vi "check unsalvageable connection.vi"(8 "error in (no error)":errorcluster, 11 "connection reference":refnum<data-value>) -> (0 "error out":errorcluster)   [LabVIEW 2015, in "SubVIs.lvlib" / "TCP Slave.lvclass"]
uses:
  <vilib>/Modbus/subvis/Protocol/TCP/TCP Slave/TCP Slave.lvclass
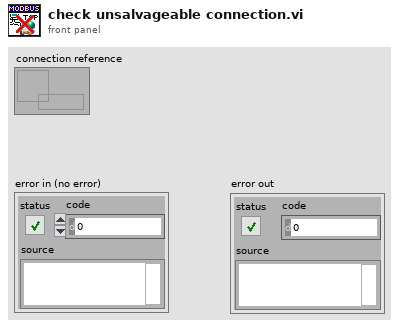
[diagram p1: front panel]
types:
  T1 = cluster{"Connected?":bool, "IP address":string, "connection error":errorcluster}
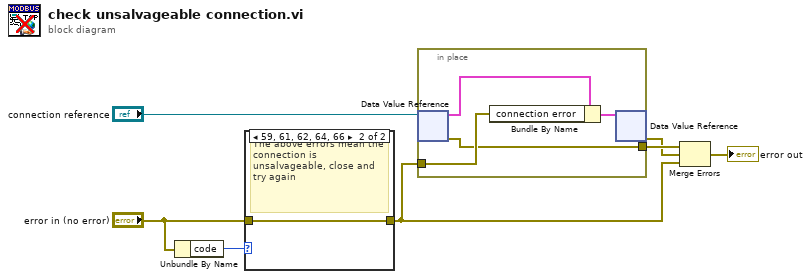
[diagram p0: block diagram]
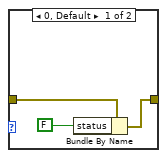
[diagram p2: hidden frame]
diagram:
  n1 = Unbundle By Name("error in (no error)") -> ("code"=w7:i32)
  n2 = case shown="59, 61, 62, 64, 66" w7 {
    tunnel: "error in (no error)" -> [w10 w11]
    tunnel: [w8 w11] -> w3
    frame 0, Default {
      n3 = Bundle By Name(cluster=w10, "status"=FALSE) -> (w8:errorcluster)
    }
    frame 59, 61, 62, 64, 66 {
      # "The above errors mean the connection is unsalvageable, close and try again"
    }
  }
  n4 = in-place {
    in-place-border: w3 -> [w13]
    in-place-border: [w12] -> w2
    n5 = in-place-dvr #1("connection reference") -> (w15:T1, w12:errorcluster)
    n6 = Bundle By Name(cluster=w15, "connection error"=w13) -> (w14:T1)
    n7 = in-place-dvr #1(w14) -> (w1:errorcluster)  [unwired: 1 out]
  }
  n8 = Merge Errors(w2, w1, w3) -> (→"error out":errorcluster)
